vi "Set Series CFG.vi"(8 "error in":errorcluster, 10 "Series CFG":string, 11 "IConfiguration UI Actor in":refnum<class "IConfiguration UI Actor.lvclass">) -> (0 "error out":errorcluster, 3 "IConfiguration UI Actor out":refnum<class "IConfiguration UI Actor.lvclass">)   [LabVIEW 2023, in "IConfiguration UI Actor.lvlib" / "IConfiguration UI Actor.lvclass"]
uses:
  IConfiguration UI Actor.lvclass
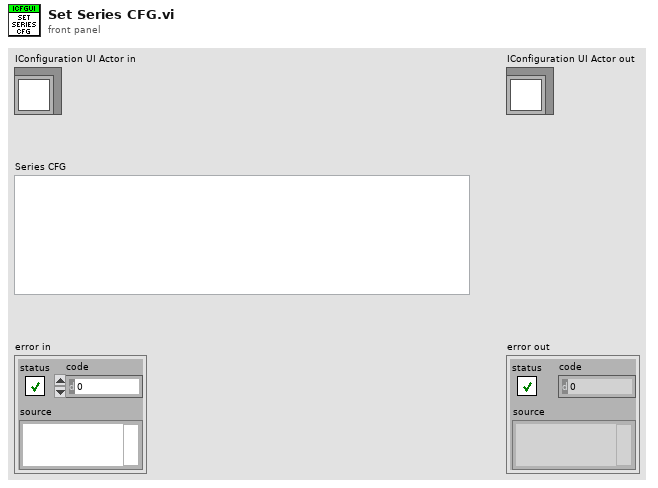
[diagram p1: front panel]
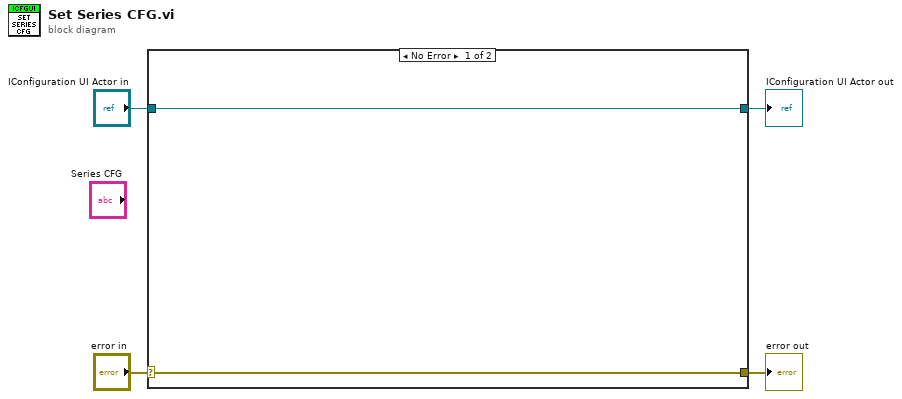
[diagram p0: block diagram]
diagram:
  n1 = case shown="No Error" "error in" {
    selector: "error in" -> [w5 w8]
    tunnel: [w5 w8] -> w3
    tunnel: [w6 w7] -> w1
    tunnel: "IConfiguration UI Actor in" -> [w6 w7]
    frame No Error {
    }
    frame Error {
    }
  }
  "error out" <- w3
  "IConfiguration UI Actor out" <- w1
